vi "FR.vi"() -> ()   [LabVIEW 2012]
uses:
  <userlib>/ImageProcessing/InitCamera_NTSC.vi
panel:
  out "Cb":dbl[][](array[numeric])
  out "Cr":dbl[][](array[numeric])
  out "y":dbl[][](array[numeric])
  out "image":picture
  in  "Stop":bool
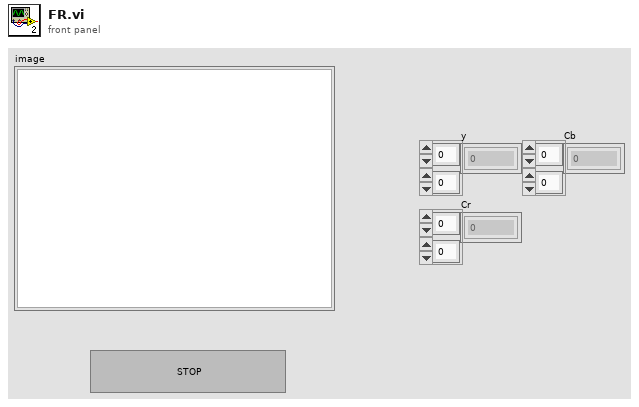
[diagram p1: front panel]
types:
  T1 = typedef "QT_Ref.ctl" = refnum<k1>
  T2 = typedef "QT_Image.ctl" = cluster{"Width":i32, "Height":i32, "Depth":i32, "data":u8[], "Compressed data":u8[], "Color table":u32[], "Duration":i32, "Options":i32, "Timestamp":i32, "ID":i32, "Reserved":i32, "Dialogs":u32}
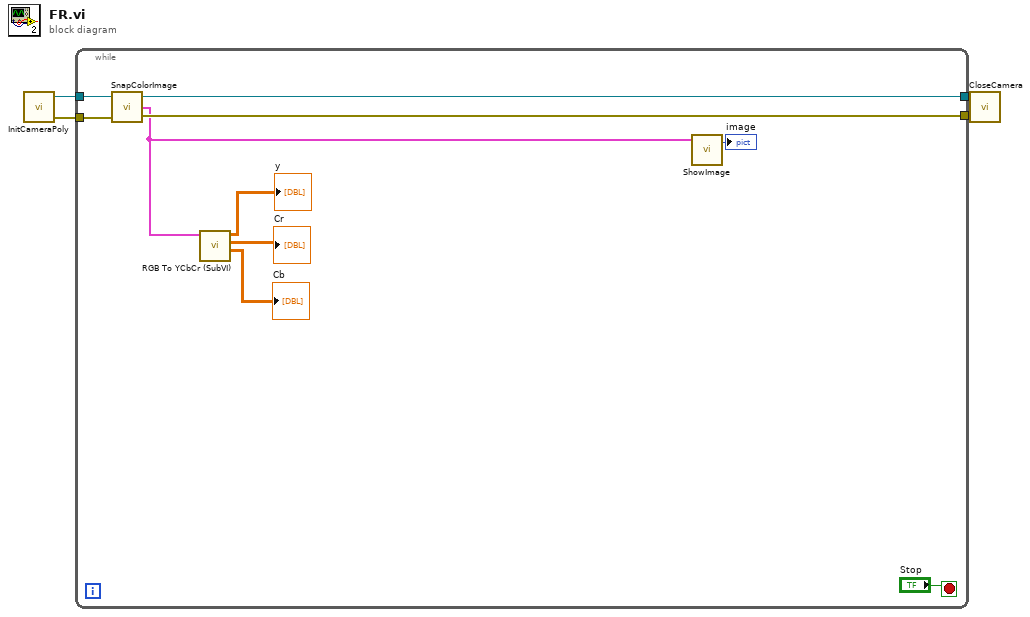
[diagram p0: block diagram]
diagram:
  n1 = call-poly <userlib>:"InitCameraPoly.vi"() -> ("error out"=w1:errorcluster, "QT Ref Out"=w2:T1)  [unwired: 2 in]
  n2 = while {
    tunnel: w1 -> [w14]
    tunnel: w2 -> [w13]
    tunnel: [w9] -> w3
    tunnel: [w12] -> w4
    stop <- "Stop" stop-if-true
    n3 = call <userlib>:"SnapColorImage.vi"("error in (no error)"=w14, "QT Ref In"=w13) -> ("error out"=w9:errorcluster, "Image Out"=w8:T2, "QT Ref Out"=w12:T1)  [unwired: 1 in]
    n4 = call "RGB To YCbCr (SubVI).vi"("Image Out"=w8) -> ("Cb"=→"Cb":dbl[][], "Cr"=→"Cr":dbl[][], "y"=→"y":dbl[][])  [unwired: 8 in]
    n5 = call <userlib>:"ShowImage.vi"("Image"=w8) -> ("image"=→"image":picture)  [unwired: 2 in, 1 out]
  }
  n6 = call <userlib>:"CloseCamera.vi"("error in (no error)"=w3, "QT Ref In"=w4) -> ()  [unwired: 1 in, 1 out]
